vi "Create (List of Model Files).vi"(8 "error in (no error)":errorcluster, 11 "Model Files":T1) -> (0 "error out":errorcluster, 3 "WeChat QR Code Detector":refnum<class "WeChat QR Code Detector.lvclass">)   [LabVIEW 2020, in "feature_detection.lvlib" / "WeChat QR Code Detector.lvclass"]
doc: "Create a WeChat QR Code Detector. This uses the WeChat Object Detection and Super Resolution Neural Networks for robust QR code detection.\n\nSpecify the path to each model file individually."
uses:
  WeChat QR Code Detector.lvclass
  Model File Paths.ctl
  WeChat QR Code Detector.lvclass/WeChat QR Code Detector.ctl
  common/bin/gartoolkit_dnn_32-1.dll
  common/common.lvlib
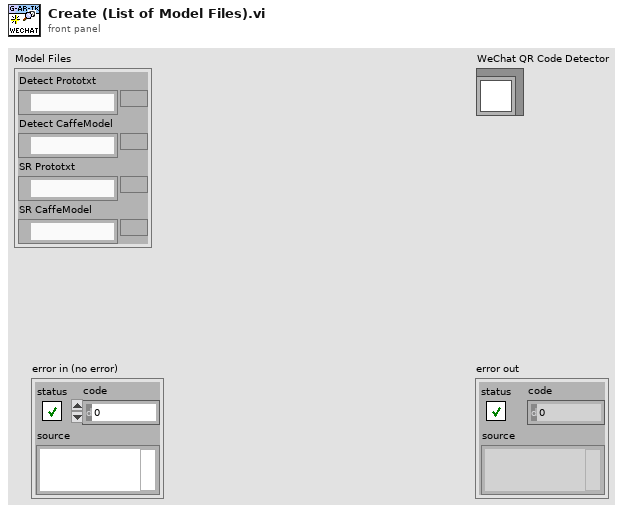
[diagram p1: front panel]
types:
  T1 = typedef "feature_detection.lvlib/WeChat QR Code Detector.lvclass/Model File Paths.ctl" = cluster{"Detect Prototxt":path, "Detect CaffeModel":path, "SR Prototxt":path, "SR CaffeModel":path}
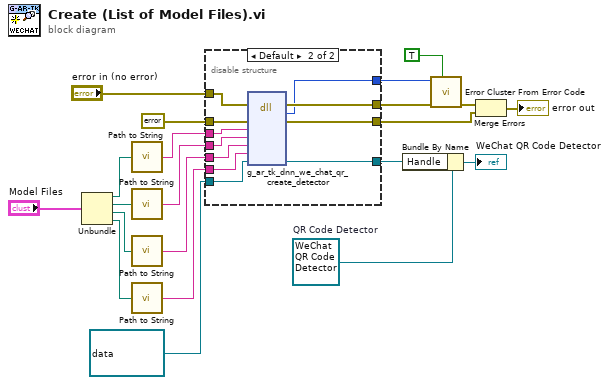
[diagram p0: block diagram]
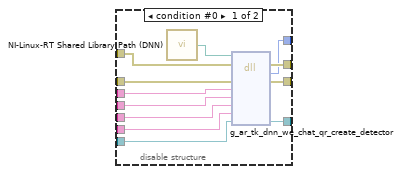
[diagram p2: hidden frame]
diagram:
  w21 = refnum<class "WeChat QR Code Detector.lvclass"> refnum  # QR Code Detector
  n1 = Unbundle("Model Files") -> ("Detect Prototxt"=w8:path, "Detect CaffeModel"=w6:path, "SR Prototxt"=w5:path, "SR CaffeModel"=w4:path)
  n2 = call "Path to String.vi"("Path"=w8) -> ("Path String"=w7:string)
  n3 = call "Path to String.vi"("Path"=w6) -> ("Path String"=w3:string)
  n4 = call "Path to String.vi"("Path"=w5) -> ("Path String"=w2:string)
  n5 = call "Path to String.vi"("Path"=w4) -> ("Path String"=w1:string)
  n6 = disable-structure shown="Default" {
    disable-tunnel: "error in (no error)" -> [w33 w44]
    disable-tunnel: errorcluster {"status"=FALSE, "code"=0, "source"=""} ("error constant") -> [w32 w43]
    disable-tunnel: w7 -> [w31 w42]
    disable-tunnel: w3 -> [w30 w41]
    disable-tunnel: w2 -> [w29 w40]
    disable-tunnel: w1 -> [w28 w39]
    disable-tunnel: refnum<data-value> refnum ("EDVR") -> [w27 w38]
    disable-tunnel: [w26 w37] -> w15
    disable-tunnel: [w25 w36] -> w14
    disable-tunnel: [w24 w35] -> w13
    disable-tunnel: [w22 w34] -> w11
    frame condition #0 {
      n7 = call "NI-Linux-RT Shared Library Path (DNN).vi"() -> ("Path"=w23:path)
      n8 = dll-call lib="?" fn="g_ar_tk_dnn_we_chat_qr_create_detector" ("g_ar_toolkit.*.*:g_ar_tk_capture_context_create")(path in=w23, error in=w33, "error_cluster"=w32, "detector_proto"=w31, "detector_model"=w30, "sr_proto"=w29, "sr_model"=w28, "EDVR"=w27) -> (error out=w26:errorcluster, w25:i32, "error_cluster"=w22:errorcluster, "EDVR"=w24:refnum<data-value>)  [unwired: 5 in, 1 out]
    }
    frame condition #1 (active) {
      n9 = dll-call lib="C:/serenial/lib/g-augmented-reality-toolkit/LabVIEW/common/bin/gartoolkit_dnn_*-1.*" fn="g_ar_tk_dnn_we_chat_qr_create_detector" ("g_ar_toolkit.*.*:g_ar_tk_capture_context_create")(error in=w44, "error_cluster"=w43, "detector_proto"=w42, "detector_model"=w41, "sr_proto"=w40, "sr_model"=w39, "EDVR"=w38) -> (error out=w37:errorcluster, "return type"=w36:i32, "error_cluster"=w34:errorcluster, "EDVR"=w35:refnum<data-value>)  [unwired: 6 in, 1 out]
    }
  }
  n10 = Bundle By Name(cluster=w21, "Handle"=w13) -> (→"WeChat QR Code Detector":refnum<class "WeChat QR Code Detector.lvclass">)
  n11 = call <vilib>:"Error Cluster From Error Code.vi"("show call chain? (False)"=TRUE, "error in (no error)"=w15, "error code (0)"=w14) -> ("error out"=w19:errorcluster)  [unwired: 6 in]
  n12 = Merge Errors(w19, w11) -> (→"error out":errorcluster)
